vi "RLC-未做相频曲线.vi"() -> ()   [LabVIEW 2021]
panel:
  out "电压比":dbl
  out "频率比":dbl
  out "频率":dbl
  out "电压2":dbl
  out "电压1":dbl
  out "XY Graph":cluster{"Y":dbl[], "Y":dbl[]}[](graph)
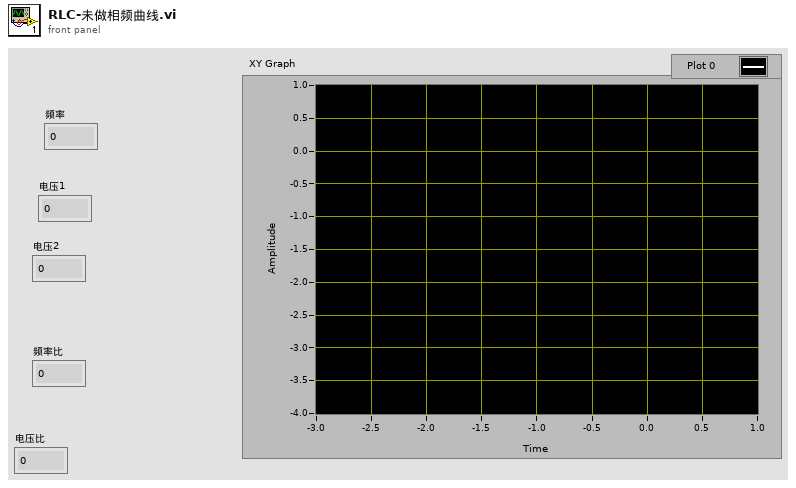
[diagram p1: front panel]
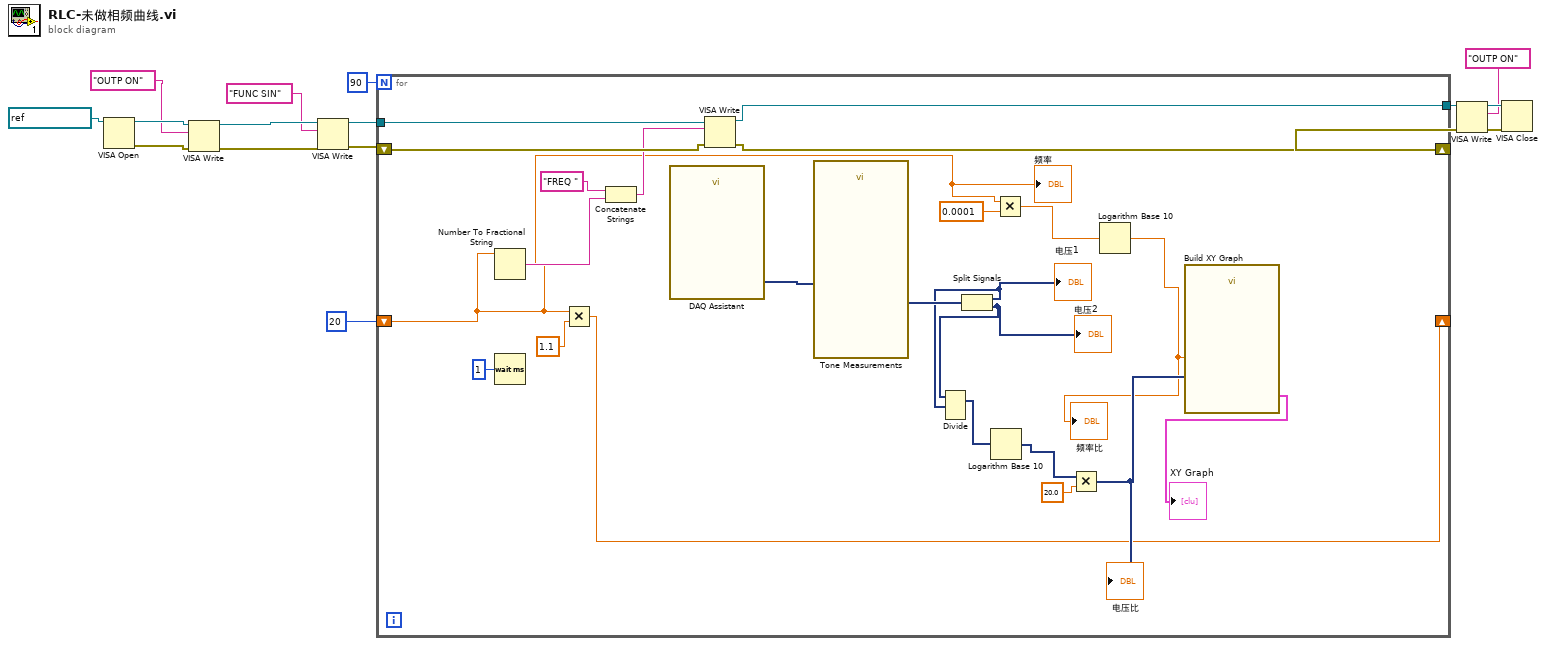
[diagram p0: block diagram]
diagram:
  n1 = VISA Open(VISA resource name=refnum<visa-resource-name> "DG1022U") -> (VISA resource name=w15:refnum<visa-resource-name>, error out=w14:errorcluster)  [unwired: 4 in]
  n2 = VISA Write(VISA resource name=w15, write buffer="OUTP ON", error in (no error)=w14) -> (VISA resource name out=w12:refnum<visa-resource-name>, error out=w10:errorcluster)  [unwired: 1 out]
  n3 = VISA Write(VISA resource name=w12, write buffer="FUNC SIN", error in (no error)=w10) -> (VISA resource name out=w6:refnum<visa-resource-name>, error out=w4:errorcluster)  [unwired: 1 out]
  n4 = for {
    N: 90 -> [_]
    tunnel: w6 -> [w39]
    tunnel: [w38] -> w5
    shift-right: [w36] -> w3
    shift-left: w4 -> [w37]
    shift-right: [w18] -> _
    shift-left: 20 -> [w17]
    n5 = Number To Fractional String(number=w17) -> (F-format string=w33:string)  [unwired: 3 in]
    n6 = Wait (ms)(milliseconds to wait=u32 1) -> ()  [unwired: 1 out]
    n7 = Multiply(x=w17, y=1.1) -> (x*y=w18:dbl)
    n8 = Concatenate Strings("FREQ " ("string"), w33) -> (w35:string)
    n9 = call "DAQ Assistant"() -> ("data"=w31:dynamicdata)  [unwired: 17 in, 2 out]
    n10 = VISA Write(VISA resource name=w39, write buffer=w35, error in (no error)=w37) -> (VISA resource name out=w38:refnum<visa-resource-name>, error out=w36:errorcluster)  [unwired: 1 out]
    n11 = call "Tone Measurements"("Signals"=w31) -> ("Amplitude"=w30:dynamicdata)  [unwired: 7 in, 3 out]
    n12 = Split Signals(w30) -> (w24:dynamicdata, w27:dynamicdata)  [unwired: 2 in]
    "电压1" <- w24
    "电压2" <- w27
    n13 = Divide(1:w24, 2:w27) -> (0:w23:dynamicdata)  [unwired: 1 in, 1 out]
    n14 = Logarithm Base 10(1:w23) -> (0:w28:dynamicdata)
    n15 = Multiply(x=w17, y=0.0001) -> (x*y=w22:dbl)
    n16 = Multiply(x=w28, y=20.0) -> (x*y=w25:dynamicdata)
    "电压比" <- w25
    n17 = Logarithm Base 10(1:w22) -> (0:w20:dbl)
    "频率比" <- w20
    n18 = call "Build XY Graph"("Y Input"=w25, "X Input"=w20) -> ("XY Graph"=→"XY Graph":cluster{"X":dbl[], "Y":dbl[]}[])  [unwired: 8 in, 1 out]
    "频率" <- w17
  }
  n19 = VISA Write(VISA resource name=w5, write buffer="OUTP ON", error in (no error)=w3) -> (VISA resource name out=w8:refnum<visa-resource-name>, error out=w9:errorcluster)  [unwired: 1 out]
  n20 = VISA Close(VISA resource name=w8, error in (no error)=w9) -> ()  [unwired: 1 out]
